vi "T-Periodic Finite Edge Tilted Top Square Gate.vi"(4 "Period T":dbl format="%#_4g", 6 "slope":dbl format="%#_4g", 8 "s_F":dbl format="%#_4g", 9 "s_R":dbl format="%#_4g", 10 "W":dbl format="%#_4g", 11 "t":dbl format="%#_4g") -> (3 "Finite Edge Square(t)":dbl format="%#_4g")   [LabVIEW 2019]
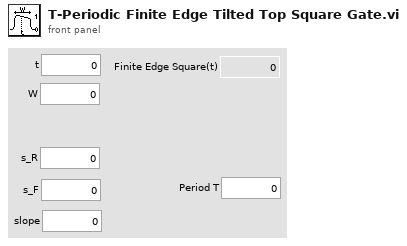
[diagram p1: front panel]
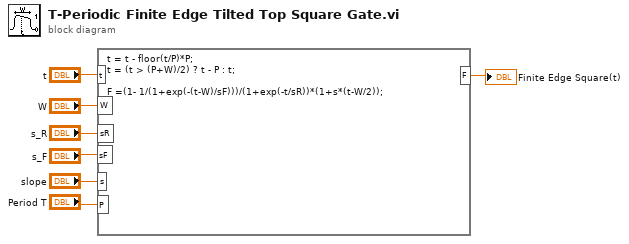
[diagram p0: block diagram]
diagram:
  n1 = formula code="t = t - floor(t/P)*P;\nt = (t > (P+W)/2) ? t - P : t;\n\nF =(1- 1/(1+exp(-(t-W)/sF)))/(1+exp(-t/sR))*(1+s*(t-W/2));"("t"="t", "W"="W", "sR"="s_R", "sF"="s_F", "s"="slope", "P"="Period T") -> ("F"=→"Finite Edge Square(t)":dbl)
